vi "fgv.vi"(7 "Get? (T)":bool=TRUE, 11 "RQMHLogger Set":refnum<class "RQMHLogger.lvclass">) -> (3 "RQMHLogger Get":refnum<class "RQMHLogger.lvclass">)   [LabVIEW 2024, in "RQMHLogSingleton.lvlib"]
uses:
  RQMHLogSingleton.lvlib
  RQMHLogger/RQMHLogger.lvclass
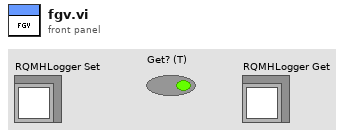
[diagram p1: front panel]
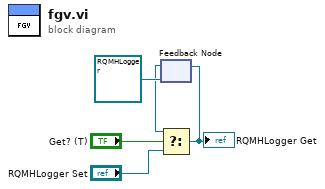
[diagram p0: block diagram]
diagram:
  n1 = feedback #1(refnum<class "RQMHLogger.lvclass"> refnum ("RQMHLogger.lvclass")) -> (w3:refnum<class "RQMHLogger.lvclass">)
  n2 = Select(t=w3, s="Get? (T)", f="RQMHLogger Set") -> (s? t:f=w1:refnum<class "RQMHLogger.lvclass">)
  "RQMHLogger Get" <- w1
  n3 = feedback-in #1(w1) -> ()
